vi "FFT Spectrum (Real-Im) for 1 Chan.vi"(4 "window parameter":dbl=nan, 6 "averaging parameters":T3={"averaging mode"=enum."No averaging", "weighting mode"=enum."Exponential", "number of averages"=10} {"number of averages" min=1}, 7 "restart averaging (F)":bool, 8 "error in (no error)":errorcluster, 10 "window":T2=1 items=["Rectangle"=0, "Hanning"=1, "Hamming"=2, "Blackman-Harris"=3, "Exact Blackman"=4, "Blackman"=5, "Flat Top"=6, "4 Term B-Harris "=7, "7 Term B-Harris"=8, "Low Sidelobe"=9, "Blackman Nuttall"=11, "Triangle"=30, "Bartlett-Hanning"=31, "Bohman"=32, "Parzen"=33, "Welch"=34, "Kaiser"=60, "Dolph-Chebyshev"=61, "Gaussian"=62], 11 "time signal":waveform(dbl)) -> (0 "error out":errorcluster, 1 "averages completed":dbl, 2 "imaginary part":T1 {"imaginary part" format="%.2p"; "f0" format="%0.2p"; "df" format="%0.2p"}, 3 "real part":cluster{"f0":dbl, "df":dbl, "real part":dbl[]} {"real part" format="%.2p"; "f0" format="%0.2p"; "df" format="%0.2p"}, 5 "averaging done":bool)   [LabVIEW 2020, in "NI_MAPro.lvlib"]
doc: "Computes the averaged FFT spectrum of <B>time signal</B>. This VI returns the FFT results as real and imaginary parts. Wire data to the <B>time signal</B> input to determine the polymorphic instance to use or manually select the instance."
uses:
  NI_MAPro.lvlib
  windowTd.ctl
  NI_AALPro.lvlib
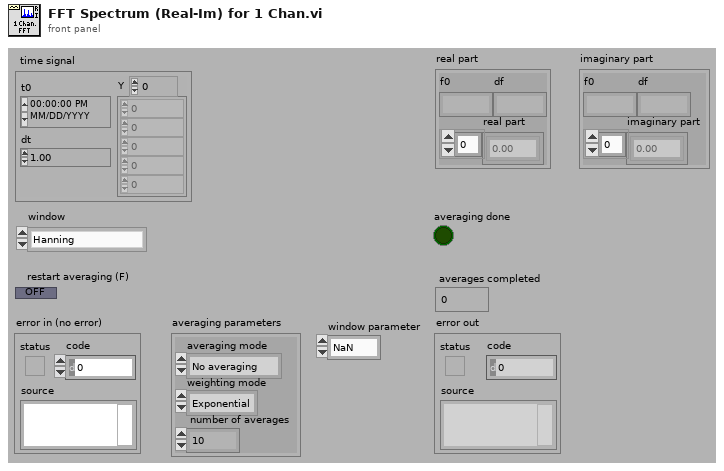
[diagram p1: front panel]
types:
  T1 = cluster{"f0":dbl, "df":dbl, "imaginary part":dbl[]}
  T2 = typedef "NI_AALPro.lvlib/windowTd.ctl" = u32
  T3 = cluster{"averaging mode":enum16{"No averaging", "Vector averaging", "RMS averaging", "Peak hold"}, "weighting mode":enum16{"Linear", "Exponential"}, "number of averages":u32}
  T4 = cluster{"block size":i32, "dt":dbl, "spectrum parameters":cluster{"averaging parameters":cluster{"averaging mode":enum16{"No averaging", "Vector averaging", "RMS averaging", "Peak hold"}, "weighting mode":enum16{"Linear", "Exponential"}, "number of averages":u32}, "window":T2}, "df":dbl, "averages completed":dbl, "complex spectrum":cdb[], "real spectrum":dbl[], "t0 history":dbl, "dt history":dbl, "timestamp":dbl, "lin avg done":bool}
  T5 = cluster{"dB On (F)":bool, "unwrap phase (F)":bool, "convert to degree (F)":bool}
  T6 = cluster{"f0":dbl, "df":dbl, "imag or phase":dbl[]}
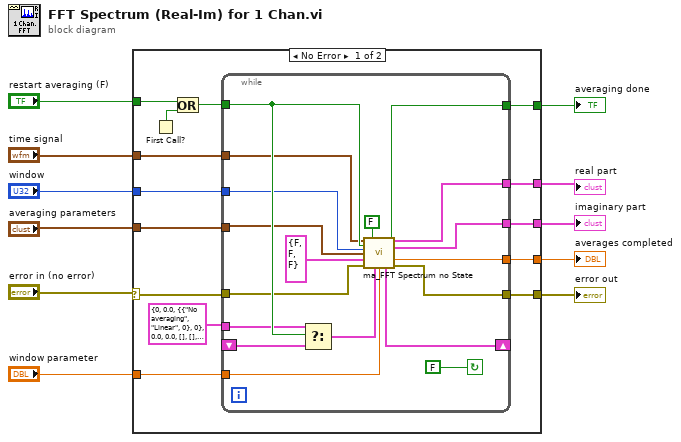
[diagram p0: block diagram]
diagram:
  n1 = case shown="No Error" "error in (no error)" {
    selector: "error in (no error)" -> [w22 w44]
    tunnel: [w23 w44] -> w11
    tunnel: "restart averaging (F)" -> [w20 _]
    tunnel: "time signal" -> [w19 _]
    tunnel: "window" -> [w18 _]
    tunnel: "averaging parameters" -> [w17 _]
    tunnel: "window parameter" -> [w16 _]
    tunnel: [w15 _] -> w4
    tunnel: [w14 _] -> w3
    tunnel: [w13 _] -> w2
    tunnel: [w12 _] -> w1
    frame No Error {
      n2 = First Call?() -> (First Call?: T/F=w25:bool)
      n3 = Or(x=w20, y=w25) -> (x .or. y?=w24:bool)
      n4 = while {
        tunnel: w18 -> [w35]
        tunnel: w22 -> [w36]
        tunnel: w19 -> [w27]
        tunnel: w17 -> [w34]
        tunnel: w24 -> [w38]
        tunnel: [w43] -> w15
        tunnel: [w42] -> w12
        tunnel: [w41] -> w14
        tunnel: [w40] -> w23
        shift-right: [w39] -> _
        shift-left: _ -> [w31]
        tunnel: T4 {"block size"=0, "dt"=0.0, "spectrum parameters"={"averaging parameters"={"averaging mode"=enum."No averaging", "weighting mode"=enum."Linear", "number of averages"=0}, "window"=0}, "df"=0.0, "averages completed"=0.0, "complex spectrum"=[], "real spectrum"=[], "t0 history"=0.0, "dt history"=0.0, "timestamp"=0.0, "lin avg done"=FALSE} ("state info") -> [w37]
        tunnel: [w29] -> w13
        tunnel: w16 -> [w26]
        stop <- FALSE continue-if-true
        n5 = Select(t=w37, s=w38, f=w31) -> (s? t:f=w32:T4)
        n6 = call "ma_FFT Spectrum no State.vi"("time signal"=w27, "restart averaging (F)"=w38, "mag-phase"=FALSE, "window"=w35, "averaging parameters"=w34, "view"=T5 {"dB On (F)"=FALSE, "unwrap phase (F)"=FALSE, "convert to degree (F)"=FALSE}, "error in"=w36, "state info"=w32, "window parameter"=w26) -> ("averaging done"=w43:bool, "real or mag"=w41:cluster{"f0":dbl, "df":dbl, "real or mag":dbl[]}, "imag or phase"=w29:T6, "averages completed"=w42:dbl, "state info"=w39:T4, "error out"=w40:errorcluster)  [unwired: 1 out]
      }
    }
    frame Error {
    }
  }
  "error out" <- w11
  "averages completed" <- w1
  "averaging done" <- w4
  "imaginary part" <- w2
  "real part" <- w3
